vi "FCScluster2SaveArray_sub.vi"(3 "Autocorrelation":cluster{dbl[], dbl[]}[](graph)) -> (1 "FCS-Data":dbl[][](array[numeric]) format="%.4f")   [LabVIEW 2009]
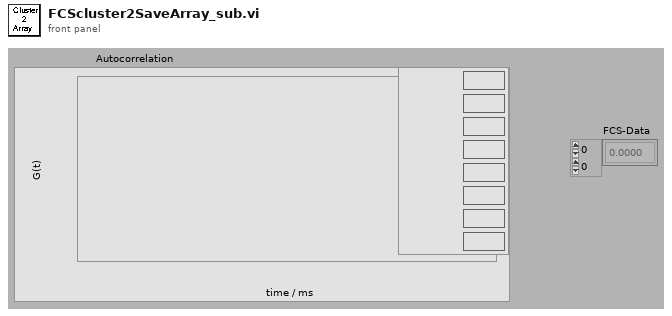
[diagram p1: front panel]
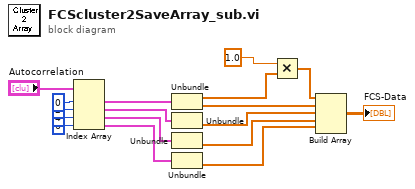
[diagram p0: block diagram]
diagram:
  n1 = Index Array(array="Autocorrelation", index #1=0 ("index"), index #2=2 ("index"), index #3=4 ("index"), index #4=6 ("index")) -> (element #1=w16:cluster{dbl[], dbl[]}, element #2=w10:cluster{dbl[], dbl[]}, element #3=w9:cluster{dbl[], dbl[]}, element #4=w8:cluster{dbl[], dbl[]})
  n2 = Unbundle(w16) -> (w2:dbl[], w15:dbl[])
  n3 = Unbundle(w10) -> (w14:dbl[])  [unwired: 1 out]
  n4 = Unbundle(w9) -> (w13:dbl[])  [unwired: 1 out]
  n5 = Unbundle(w8) -> (w12:dbl[])  [unwired: 1 out]
  n6 = Multiply(x=1.0, y=w2) -> (x*y=w1:dbl[])
  n7 = Build Array(w1, w15, w14, w13, w12) -> (→"FCS-Data":dbl[][])
